vi "Step Core.vi"(8 "error in (no error)":errorcluster, 11 "SPECAN_PVT in":refnum<class "SPECAN_PVT.lvclass">) -> (0 "error out":errorcluster, 3 "SPECAN_PVT out":refnum<class "SPECAN_PVT.lvclass">)   [LabVIEW 2018, in "SPECAN_PVT.lvlib" / "SPECAN_PVT.lvclass"]
uses:
  SPECAN_PVT.lvclass
  Plugins/Measurement Interface.lvlibp/Measurement Interface.lvclass
  C:/Sequence Automation/Plugins/Measurement Interface.lvlibp/Measurement Interface.lvclass
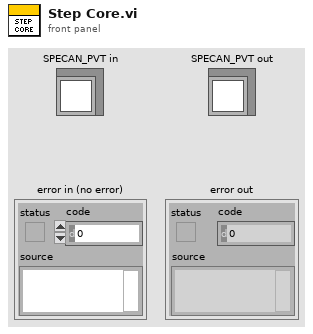
[diagram p1: front panel]
types:
  T1 = typedef "TestStand API Tools (TSAT).lvlibp/TSAT Evaluation Actions.lvlib/TSAT Evaluation.ctl" = cluster{"Test Name":string, "Pin":string, "Units":string, "SI Scaling":T2, "Test Number":i32, "Published Data Id":string, "Low Limit":dbl, "High Limit":dbl, "Export Data Location":string, "Software Bin":i64, "Evaluation Type":T3, "Test Data Source":string}
  T2 = typedef "TestStand API Tools (TSAT).lvlibp/TSAT Evaluation Actions.lvlib/TSAT Eval SI Unit Scaling.ctl" = i16
  T3 = typedef "TestStand API Tools (TSAT).lvlibp/TSAT Evaluation Actions.lvlib/TSAT Evaluation Type.ctl" = enum16{"Numeric Limit", "Pass/Fail", "None"}
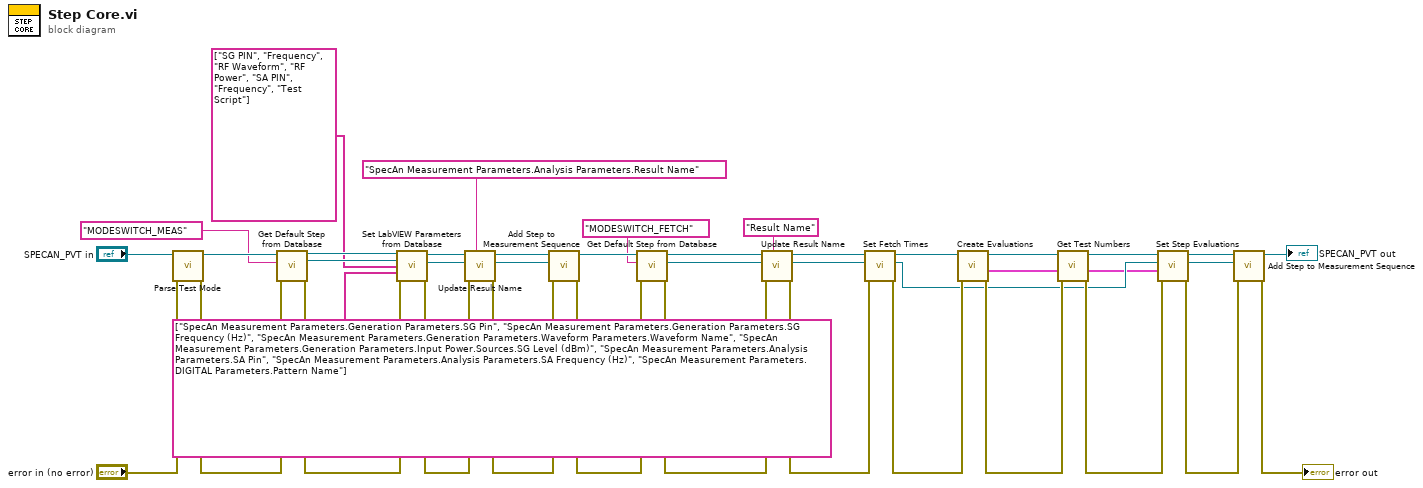
[diagram p0: block diagram]
diagram:
  n1 = call-dynamic "Parse Test Mode.vi"("error in (no error)"="error in (no error)", "SPECAN_PVT in"="SPECAN_PVT in") -> ("error out"=w38:errorcluster, "SPECAN_PVT out"=w39:refnum<class "SPECAN_PVT.lvclass">)  [unwired: 8 in]
  n2 = call "Get Default Step from Database.vi"("error in (no error)"=w38, "Default Step"="MODESWITCH_MEAS", "Measurement Interface in"=w39) -> ("error out"=w36:errorcluster, "Cloned Step"=w34:refnum<k7>, "Measurement Interface out"=w37:refnum<class "SPECAN_PVT.lvclass">)  [unwired: 6 in]
  n3 = call "Set LabVIEW Parameters from Database.vi"("Measurement Interface in"=w37, "Step In"=w34, "Dictionary Keys"=string[] ["SG PIN", "Frequency", "RF Waveform", "RF Power", "SA PIN", "Frequency", "Test Script"], "LabVIEW Parameter Mapping"=string[] ["SpecAn Measurement Parameters.Generation Parameters.SG Pin", "SpecAn Measurement Parameters.Generation Parameters.SG Frequency (Hz)", "SpecAn Measurement Parameters.Generation Parameters.Waveform Parameters.Waveform Name", "SpecAn Measurement Parameters.Generation Parameters.Input Power.Sources.SG Level (dBm)", "SpecAn Measurement Parameters.Analysis Parameters.SA Pin", "SpecAn Measurement Parameters.Analysis Parameters.SA Frequency (Hz)", "SpecAn Measurement Parameters.DIGITAL Parameters.Pattern Name"], "error in (no error)"=w36) -> ("Measurement Interface out"=w31:refnum<class "SPECAN_PVT.lvclass">, "Step Out"=w29:refnum<k7>, "error out"=w30:errorcluster)  [unwired: 8 in]
  n4 = call-dynamic "Update Result Name.vi"("LV Result Name Property"="SpecAn Measurement Parameters.Analysis Parameters.Result Name", "error in (no error)"=w30, "Step In"=w29, "SPECAN_PVT in"=w31) -> ("error out"=w27:errorcluster, "Step Out"=w24:refnum<k7>, "SPECAN_PVT out"=w28:refnum<class "SPECAN_PVT.lvclass">)  [unwired: 5 in]
  n5 = call "Add Step to Measurement Sequence.vi"("error in (no error)"=w27, "Step to Add"=w24, "Measurement Interface in"=w28) -> ("error out"=w25:errorcluster, "Measurement Interface out"=w26:refnum<class "SPECAN_PVT.lvclass">)  [unwired: 7 in]
  n6 = call "Get Default Step from Database.vi"("error in (no error)"=w25, "Default Step"="MODESWITCH_FETCH", "Measurement Interface in"=w26) -> ("error out"=w18:errorcluster, "Cloned Step"=w17:refnum<k7>, "Measurement Interface out"=w19:refnum<class "SPECAN_PVT.lvclass">)  [unwired: 6 in]
  n7 = call-dynamic "Update Result Name.vi"("LV Result Name Property"="Result Name", "error in (no error)"=w18, "Step In"=w17, "SPECAN_PVT in"=w19) -> ("error out"=w15:errorcluster, "Step Out"=w14:refnum<k7>, "SPECAN_PVT out"=w16:refnum<class "SPECAN_PVT.lvclass">)  [unwired: 5 in]
  n8 = call-dynamic "Set Fetch Times.vi"("error in (no error)"=w15, "Fetch Step In"=w14, "SPECAN_PVT in"=w16) -> ("error out"=w6:errorcluster, "Step Out"=w4:refnum<k7>, "SPECAN_PVT out"=w8:refnum<class "SPECAN_PVT.lvclass">)  [unwired: 6 in]
  n9 = call-dynamic "Create Evaluations.vi"("error in (no error)"=w6, "SPECAN_PVT in"=w8) -> ("error out"=w11:errorcluster, "Evaluations Out"=w2:T1[], "SPECAN_PVT out"=w12:refnum<class "SPECAN_PVT.lvclass">)  [unwired: 7 in]
  n10 = call-dynamic "Get Test Numbers.vi"("error in (no error)"=w11, "Evaluations In"=w2, "SPECAN_PVT in"=w12) -> ("error out"=w9:errorcluster, "Evaluations Out"=w1:T1[], "SPECAN_PVT out"=w10:refnum<class "SPECAN_PVT.lvclass">)  [unwired: 6 in]
  n11 = call-dynamic "Set Step Evaluations.vi"("error in (no error)"=w9, "Evaluation Data"=w1, "Step In"=w4, "SPECAN_PVT in"=w10) -> ("error out"=w5:errorcluster, "Step out"=w3:refnum<k7>, "SPECAN_PVT out"=w7:refnum<class "SPECAN_PVT.lvclass">)  [unwired: 5 in]
  n12 = call "Add Step to Measurement Sequence.vi"("error in (no error)"=w5, "Step to Add"=w3, "Measurement Interface in"=w7) -> ("error out"=→"error out":errorcluster, "Measurement Interface out"=→"SPECAN_PVT out":refnum<class "SPECAN_PVT.lvclass">)  [unwired: 7 in]
